vi "HW_GEN_Construct Initial VCH Modu Configuration.vi"(8 "error in":errorcluster, 9 "VCHmodu":T2, 10 "ModCFG in":T1[](array[typedef]), 11 "VarList":cluster{"Tag":string[], "Name":string[]}) -> (0 "error out":errorcluster, 2 "ModCFG to File":T1[](array[typedef]), 3 "ModuCFG out":T1)   [LabVIEW 2016]
uses:
  Gantner/HW_Module Info.ctl
  Ctrls/HardWare Basic Info _ Channel.ctl
  Ctrls/HardWare _ Module Configuration.ctl
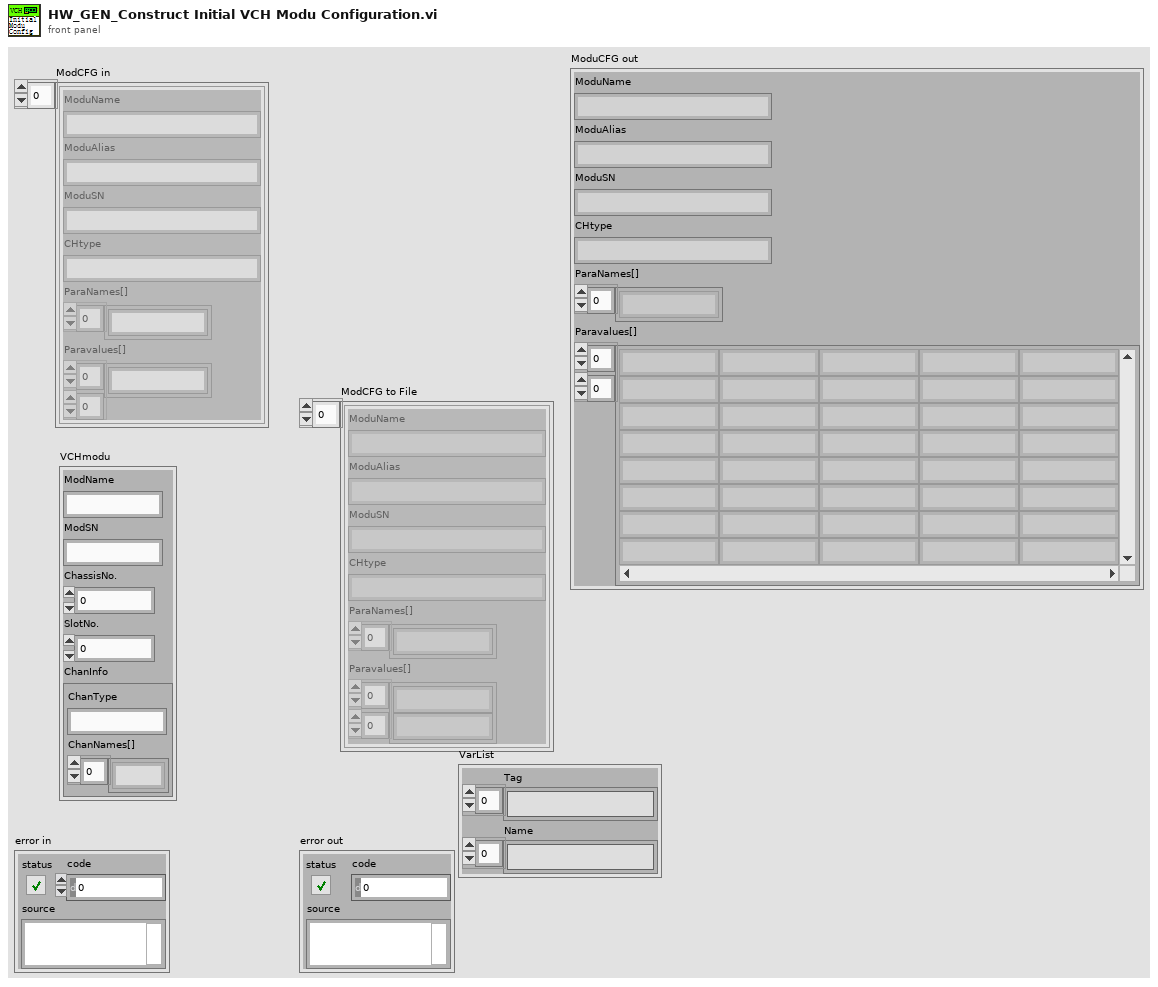
[diagram p1: front panel]
types:
  T1 = typedef "HardWare _ Module Configuration.ctl" = cluster{"ModuName":string, "ModuAlias":string, "ModuSN":string, "CHtype":string, "ParaNames[]":string[], "Paravalues[]":string[][]}
  T2 = typedef "HW_Module Info.ctl" = cluster{"ModName":string, "ModSN":string, "ChassisNo.":u32, "SlotNo.":u32, "ChanInfo":T3}
  T3 = typedef "HardWare Basic Info _ Channel.ctl" = cluster{"ChanType":string, "ChanNames[]":string[]}
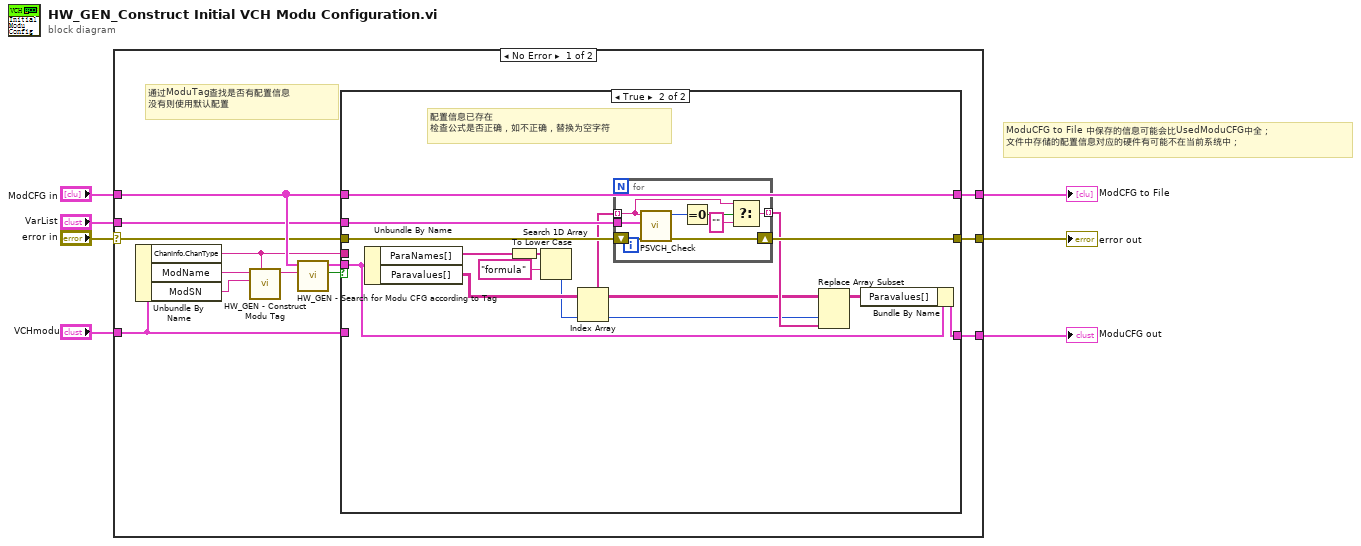
[diagram p0: block diagram]
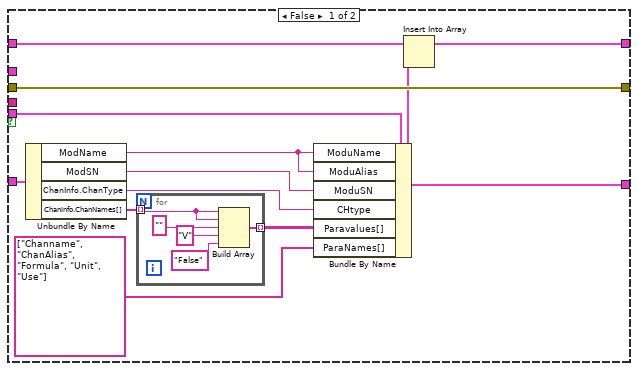
[diagram p2: hidden frame]
diagram:
  # "ModuCFG to File 中保存的信息可能会比UsedModuCFG中全；\n文件中存储的配置信息对应的硬件有可能不在当前系统中；"
  n1 = case shown="No Error" "error in" {
    selector: "error in" -> [w15 w60]
    tunnel: "VCHmodu" -> [w20 _]
    tunnel: [w19 _] -> w6
    tunnel: [w18 _] -> w5
    tunnel: [w17 w60] -> w4
    tunnel: "ModCFG in" -> [w16 _]
    tunnel: "VarList" -> [w8 _]
    frame No Error {
      # "通过ModuTag查找是否有配置信息\n没有则使用默认配置"
      n2 = Unbundle By Name(w20) -> ("ChanInfo.ChanType"=w9:string, "ModName"=w11:string, "ModSN"=w10:string)
      n3 = call "HW_GEN - Construct Modu Tag.vi"("ChanType"=w9, "ModSN"=w10, "ModName"=w11) -> ("String"=w12:string)  [unwired: 8 in]
      n4 = call "HW_GEN - Search for Modu CFG according to Tag.vi"("ModuTag"=w12, "ModuCFG[]"=w16) -> ("find?"=w14:bool, "ModuCFG out"=w13:T1)  [unwired: 7 in, 1 out]
      n5 = case shown="True" w14 {
        tunnel: w15 -> [w32 w49]
        tunnel: w13 -> [w29 w47]
        tunnel: [w21 w39] -> w19
        tunnel: [w32 w48] -> w17
        tunnel: w16 -> [w31 w51]
        tunnel: [w30 w51] -> w18
        tunnel: w20 -> [w28 _]
        tunnel: w9 -> [_ _]
        tunnel: w8 -> [_ w50]
        frame False {
          n6 = Unbundle By Name(w28) -> ("ModName"=w27:string, "ModSN"=w26:string, "ChanInfo.ChanType"=w25:string, "ChanInfo.ChanNames[]"=w24:string[])
          n7 = for {
            tunnel: w24 -> [w37] mode=indexing
            tunnel: [w33] -> w22 mode=indexing
            n8 = Build Array(w37, w37, "", "V" ("element"), "False" ("element")) -> (w33:string[])
          }
          n9 = Bundle By Name(cluster=w29, "ModuName"=w27, "ModuAlias"=w27, "ModuSN"=w26, "CHtype"=w25, "Paravalues[]"=w22, "ParaNames[]"=string[] ["Channame", "ChanAlias", "Formula", "Unit", "Use"] ("DisCols[]")) -> (w21:T1)
          n10 = Insert Into Array(array=w31, new element=w21) -> (w30:T1[])  [unwired: 1 in]
        }
        frame True {
          # "配置信息已存在\n检查公式是否正确，如不正确，替换为空字符"
          n11 = Unbundle By Name(w47) -> ("ParaNames[]"=w46:string[], "Paravalues[]"=w41:string[][])
          n12 = To Lower Case(string=w46) -> (all lower case string=w45:string[])
          n13 = Search 1D Array(1D array=w45, element="formula") -> (index of element=w40:i32)  [unwired: 1 in]
          n14 = Index Array(array=w41, index (col)=w40) -> (element=w43:string[])  [unwired: 1 in]
          n15 = for {
            tunnel: w50 -> [w59]
            shift-right: [w57] -> w48
            shift-left: w49 -> [w58]
            tunnel: w43 -> [w54] mode=indexing
            tunnel: [w52] -> w42 mode=indexing
            n16 = call "PSVCH_Check.vi"("Error In (no error)"=w58, "VarList"=w59, "Formula"=w54) -> ("Error Out"=w57:errorcluster, "code"=w56:i32)  [unwired: 4 in, 3 out]
            n17 = Equal To 0?(x=w56) -> (x = 0?=w55:bool)
            n18 = Select(t=w54, s=w55, f="") -> (s? t:f=w52:string)
          }
          n19 = Replace Array Subset(array=w41, new element=w42, index (col)=w40) -> (w38:string[][])  [unwired: 1 in]
          n20 = Bundle By Name(cluster=w47, "Paravalues[]"=w38) -> (w39:T1)
        }
      }
    }
    frame Error {
    }
  }
  "ModuCFG out" <- w6
  "ModCFG to File" <- w5
  "error out" <- w4
